vi "MoveRel_all.vi"(7 "# axis":i32, 8 "error in (no error)":errorcluster, 10 "Position":dbl[](array[numeric]), 11 "VISA resource name":refnum<visa-resource-name>) -> (0 "error out":errorcluster)   [LabVIEW 2012, in "Micos_uic.lvlib"]
doc: "Performs an instrument error query before terminating the software connection to the instrument."
uses:
  Micos_uic.lvlib
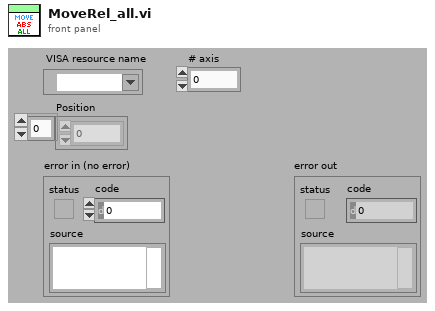
[diagram p1: front panel]
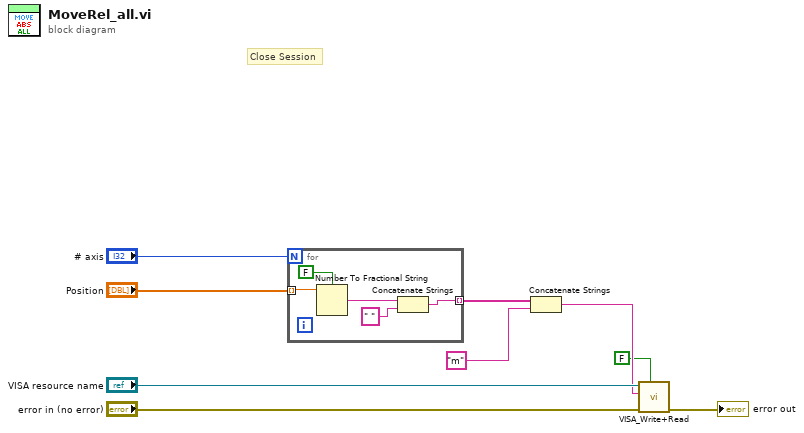
[diagram p0: block diagram]
diagram:
  # "Close Session"
  n1 = for {
    N: "# axis" -> [_]
    tunnel: "Position" -> [w14] mode=indexing
    tunnel: [w10] -> w5 mode=indexing
    n2 = Number To Fractional String(use system decimal point (T)=FALSE, number=w14) -> (F-format string=w12:string)  [unwired: 2 in]
    n3 = Concatenate Strings(w12, " " ("string")) -> (w10:string)
  }
  n4 = Concatenate Strings(w5, "m" ("format string")) -> (w2:string)
  n5 = call "VISA_Write+Read.vi"("Read?"=FALSE, "error in (no error)"="error in (no error)", "Write Buffer"=w2, "VISA resource name"="VISA resource name") -> ("error out"=→"error out":errorcluster)  [unwired: 5 in, 2 out]
